vi "CSM_creep_function.vi"() -> ()   [LabVIEW 2009]
doc: "This is the sample data playback waveform and data logging example program. Sample data points are generated using MX Sample Data Array Generator.vi. You will need to replace this VI with your own code. New sample data is sent to the controller each time a status message is recieved from the controller that the next random buffer is running.\nThis program also shows you how to use Active X events. These are used to notify the program when a data buffer is ready for collection and when to load a new buffer of sample data points. Two separate event queues are used: one for data logging and the other for general status, such as when a sample data point buffer can be sent to the controller. Each event handler must run in parallel loops as execution passes to MX Handle Status Change Event.vi and MX Handle Data Ready Event.vi and will not come out of them until an event is received from the console program. When modifiying this example for your own use you may want to setup a third loop to be doing other processing, or you could add code to manipulate the data buffer in the data monitoring loop."
panel:
  in  "Maximum Value":dbl[](array[numeric]) format="%.2f"
  out "Units Strings":string[](array[string])
  in  "Control Modes":u16[](array[ring])=[0, 0, 0, 0] items=["Channel 1", "Channel 2", "Channel 3", "Channel 4"]
  out "Waveform Graph":dbl[][](graph)
  in  "Number of Columns":i32[](array[numeric])
  in  "Interval/Buffer Parameters":T1={"Sample interval - ms (2)"=2.0, "Buffer Length (1000)"=1000, "No. of Buffers (0)"=0} {"Sample interval - ms (2)" min=0.2 format="%.1f"}
  in  "Column Types":i32[][](array[ring])=[[0, 0, 0, 0, 0, 0, 0, 0]] items=["Feedback", "Direct Auxillary"]
  in  "Column Channels":i32[][](array[numeric])=[[1, 1, 1, 1, 1, 1, 1, 1]] min=0 max=200
  in  "Start/Stop":bool
  in  "Axis Selector":i32[](listbox)
  # "Axis 1\nAxis 2\nAxis 3\nAxis 4"
  # "Axis 1\nAxis 2\nAxis 3\nAxis 4"
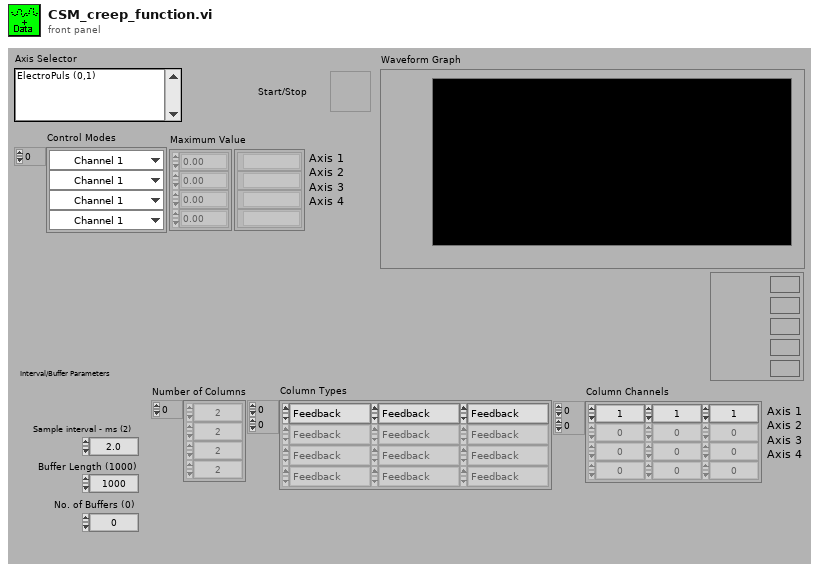
[diagram p1: front panel]
types:
  T1 = cluster{"Sample interval - ms (2)":dbl, "Buffer Length (1000)":i32, "No. of Buffers (0)":i32}
  T2 = cluster{"Name":string, "Type":i32, "SI Full Scale":dbl, "Full Scale":dbl, "Units String":string, "Display Format":string, "Gauge Length":dbl}[][]
  T3 = cluster{"Device ID":i32, "Device Name":string, "Device Type":i32}[]
  T4 = cluster{"Data Sample Format (0)":i8, "Loop code (2)":i8, "Target Amplitude (32767)":i16, "Playback rate":dbl, "Playback Scale":dbl[], "Envelope Ramp Rate":dbl, "Filter Order (0)":i8, "Filter Type (0)":i8, "Filter Bandwidth":dbl}
  T5 = typedef "System Status Reports.ctl" = enum16{"Not this device", "Not Recognised", "Ramp Stopped", "Ramp Running", "Ramp Held", "Random Stopped", "Random Held", "Load Random", "Load Sample", "Sample Playback Held", "Sample Playback Stop - Buffer Underrun", "Sample Playback Continuing", "Returning - EM Frame", "Error Trip", "Segment Counter Trip", "Cycle Counter Trip", "Limit Trip", "Cyclic Stopped", "Cyclic running", "Cyclic Held", "Cyclic Finishing", "Analogue Event 1 tripped", "Analogue Event 2 tripped", "Analogue Event 3 tripped", "Analogue Event 4 tripped", "Analogue Event Off, prepared, armed", "Digital Event Tripped", "Digital Event Off, Prepared, Armed", "Grips Open", "Crosshead Unclamped", "Pump Power Off", "Actuator not Active", "Fault", "Calibrated", "Calibration/Balance in progress", "Console Stop Button Pressed", "Control mode change", "Set Point Change", "Transducer Over-ranged", "GPIB Trigger Armed", "GPIB Trigger Tripped", "Group Trigger Event Tripped", "Trimodal Control Saturated", "Trimodal Control Peak Error", "Trimodal Peak Not Updating", "Digital Line Low", "Digital Line High", "Transducer Disconnected", "Transducer Connected", "Data Logger Idle", "Data Logger Stopped", "Data Logger Started", "Data Logger Data Overrun", "Sample Data Playback Event Tripped", "Next Control Mode Change", "Autotune Completed OK", "Autotune Failed", "Motor Maximum Power Exceeded", "Motor Maximum Temperature Too High", "Motor Maximum Power & Temp too high", "Button Pressed - Function 1", "Button Pressed - Function 2", "Button Pressed - Specimen Protect", "Button Pressed - Reset Gauge Length", "Button Pressed - Return", "Button Pressed - Stop", "Button Pressed - Start", "1st Tensile Travel Limit Tripped", "1st Compressive Travel Limit Tripped", "2nd Tensile Travel Limit Tripped", "2nd Compressive Travel Limit Tripped", "Frame Relay Power Fault - EM", "Emergency Stop - EM", "Drive Disabled - EM", "Power Amp Fault - EM", "Motor Over-Temperature Fault - EM", "Top Grip Open - EM", "Bottom Grip Open - EM", "Interlock Active - EM", "PIP Button Pushed - EM", "Close Grip Request - EM", "High Clutch Active - EM", "Crosshead Moving - EM"}
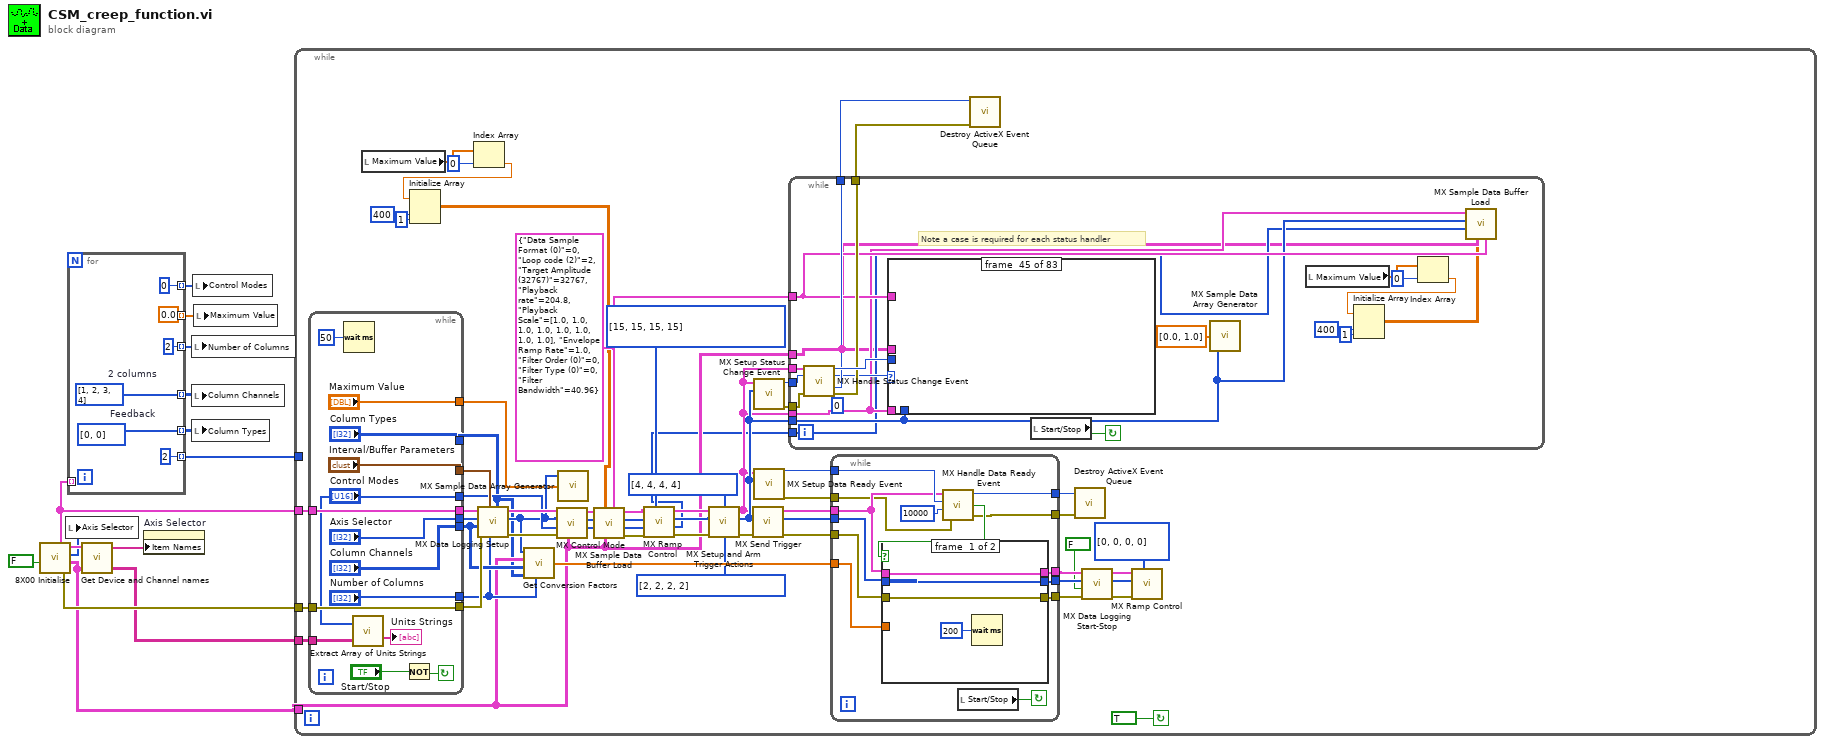
[diagram p0: block diagram]
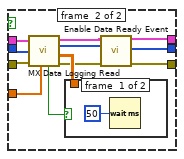
[diagram p2: hidden frame]
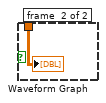
[diagram p3: hidden frame]
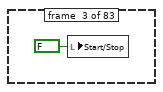
[diagram p6: hidden frame]
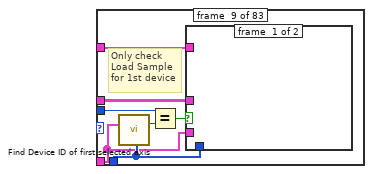
[diagram p12: hidden frame]
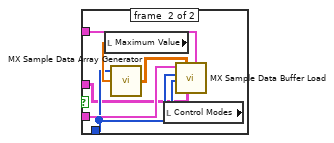
[diagram p13: hidden frame]
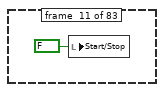
[diagram p15: hidden frame]
diagram:
  n1 = call "8X00 Initialise.vi"("Reset?"=FALSE ("Reset")) -> ("error out"=w12:errorcluster, "Channel Data"=w9:T2, "Axis Selector"=w2:i32[], "Axis Information"=w7:T3)  [unwired: 3 in]
  n2 = local write "Axis Selector"(w2) -> ()
  n3 = for {
    tunnel: w7 -> [_] mode=indexing
    tunnel: [w19] -> w11 mode=indexing
    tunnel: [w18] -> w10 mode=indexing
    tunnel: [2] -> w8 mode=indexing
    tunnel: [2] -> w5 mode=indexing
    tunnel: [0.0] -> w4 mode=indexing
    tunnel: [0] -> w3 mode=indexing
    w18 = i32[] [0, 0]  # Feedback
    w19 = i32[] [1, 2, 3, 4]  # 2 columns
  }
  n4 = call "Get Device and Channel names.vi"("Axis Information"=w7, "Channel Data"=w9) -> ("Device Names"=w13:string[], "Units Strings"=w6:string[][])  [unwired: 1 out]
  n5 = property on="Axis Selector" class="ListBox (strict)"("Item Names"=w13) -> ()  [unwired: 2 in, 2 out]
  n6 = local write "Number of Columns"(w5) -> ()
  n7 = local write "Column Channels"(w11) -> ()
  n8 = local write "Column Types"(w10) -> ()
  n9 = local write "Control Modes"(w3) -> ()
  n10 = local write "Maximum Value"(w4) -> ()
  n11 = while {
    tunnel: w6 -> [w44]
    tunnel: w8 -> [_]
    tunnel: w9 -> [w29]
    tunnel: w7 -> [w75]
    tunnel: w12 -> [w78]
    stop <- TRUE continue-if-true
    w28 = T4 {"Data Sample Format (0)"=0, "Loop code (2)"=2, "Target Amplitude (32767)"=32767, "Playback rate"=204.8, "Playback Scale"=[1.0, 1.0, 1.0, 1.0, 1.0, 1.0, 1.0, 1.0], "Envelope Ramp Rate"=1.0, "Filter Order (0)"=0, "Filter Type (0)"=0, "Filter Bandwidth"=40.96} ("Sample Data Playback Definition")
    w36 = u16[] [0, 0, 0, 0] items=["Stop", "Start or continue", "Hold", "Continue", "Return ramp to set level at fixed rate", "Reserved", "Reserved", "Start Random without demand hold", "Start Random with demand hold", "Prepare Random Start without demand hold", "Prepare Random Start with demand hold", "Unslave", "Reserved", "Reserved", "Start Sample Data Playback or Resume", "Prepare for Start of Sample Data", "Reserved", "Reserved", "Resume Playback"] ("Ramp Control")
    w40 = u16[] [15, 15, 15, 15] items=["Stop", "Start or continue", "Hold", "Continue", "Return ramp to set level at fixed rate", "Reserved", "Reserved", "Start Random without demand hold", "Start Random with demand hold", "Prepare Random Start without demand hold", "Prepare Random Start with demand hold", "Unslave", "Reserved", "Reserved", "Start Sample Data Playback or Resume", "Prepare for Start of Sample Data", "Reserved", "Reserved", "Resume Playback"] ("Ramp Control")
    w61 = u16[] [2, 2, 2, 2] items=["None", "Stop Data Logging", "Start Data Logging"] ("Remote Trigger Action - Data Logging")
    w66 = u16[] [4, 4, 4, 4] items=["None", "Actuator Off", "Stop Waveform", "Hold Waveform", "Transfer", "Log Data Point", "Reset Waveform"] ("Remote Trigger Action")
    # "Note a case is required for each status handler"
    n12 = while {
      tunnel: ["Maximum Value"] -> w42
      tunnel: w44 -> [w83]
      tunnel: ["Control Modes"] -> w45
      tunnel: ["Number of Columns"] -> w72
      tunnel: ["Interval/Buffer Parameters"] -> w76
      tunnel: ["Column Types"] -> w27
      tunnel: [w91] -> w77
      tunnel: w78 -> [w91]
      tunnel: ["Column Channels"] -> w74
      tunnel: ["Axis Selector"] -> w79
      tunnel: [w94] -> w80
      tunnel: w75 -> [w94]
      stop <- w90 continue-if-true
      n13 = Wait (ms)(milliseconds to wait=u32 50) -> ()  [unwired: 1 out]
      n14 = call "Extract Array of Units Strings.vi"("Axes Units Strings"=w83, "Control Modes"="Control Modes") -> ("Units Strings"=→"Units Strings":string[])
      n15 = Not(x="Start/Stop") -> (.not. x?=w90:bool)
    }
    n16 = local read "Maximum Value"() -> (w23:dbl[])
    n17 = Index Array(array=w23, index=0) -> (element=w22:dbl)
    n18 = Initialize Array(w22, 400 ("dimension size"), 1 ("dimension size")) -> (w20:dbl[][])
    n19 = call "MX Data Logging Setup.vi"("Column Types"=w27, "Number of Columns"=w72, "Interval/Buffer Parameters"=w76, "error in (no error)"=w77, "Column Channels"=w74, "Axis Selector"=w79, "Axis Information"=w80) -> ("error out"=w50:errorcluster, "Axis Selector copy"=w43:i32[], "Axis Information out"=w49:T3)  [unwired: 1 out]
    n20 = call "Get Conversion Factors.vi"("Axis Selector"=w43, "Channel Data"=w29, "Column Channels"=w74, "Column Types"=w27, "Number of Columns"=w72) -> ("Conversion Factors"=w73:dbl[])
    n21 = call "MX Control Mode.vi"("Channel Data"=w29, "error in (no error)"=w50, "Control Modes"=w45, "Axis Selector"=w43, "Axis Information"=w49) -> ("Control Modes out"=w46:u16[], "Axis Selector out"=w47:i32[], "Axis Information out"=w48:T3)  [unwired: 1 in, 1 out]
    n22 = call "MX Sample Data Array Generator.vi"("Maximum Value"=w42, "Axis Selector"=w43) -> ()  [unwired: 1 in, 1 out]
    n23 = call "MX Sample Data Buffer Load.vi"("Sample Data Playback Definition"=w28, "Channel Data"=w29, "Sample Data"=w20, "Channels In"=w46, "Axis Selector In"=w47, "Axis Information In"=w48) -> ("error out"=w52:errorcluster, "Channels Out"=w41:u16[], "Axis Selector Out"=w54:i32[], "Axis Information Out"=w56:T3)  [unwired: 2 in]
    n24 = call "MX Ramp Control.vi"("Ramp Control"=w40, "error in (no error)"=w52, "Channels In"=w41, "Axis Selector In"=w54, "Axis Information In"=w56) -> ("error out"=w51:errorcluster, "Channels Out"=w26:u16[], "Axis Selector Out"=w53:i32[], "Axis Information Out"=w55:T3)  [unwired: 2 in]
    n25 = call "MX Setup and Arm Trigger Actions.vi"("Remote Trigger Action"=w66, "Axis Information In"=w55, "Axis Selector"=w53, "Remote Trigger Action - Data Logging"=w61, "error in (no error)"=w51) -> ("Axis Information Out"=w30:T3, "Axis Selector copy"=w33:i32[], "error out"=w62:errorcluster)  [unwired: 2 in]
    n26 = call "MX Send Trigger.vi"("error in (no error)"=w62, "Axis Selector"=w33, "Axis Information"=w30) -> ("error out"=w64:errorcluster, "Axis Selector copy"=w63:i32[], "Axis Information out"=w65:T3)  [unwired: 2 in]
    n27 = call "MX Setup Status Change Event.vi"("Axis Selector"=w33, "Axis Information"=w30) -> ("error out"=w34:errorcluster, "Event Queue"=w35:u32)  [unwired: 6 in]
    n28 = call "MX Setup Data Ready Event.vi"("Axis Selector"=w33, "Axis Information"=w30) -> ("Error Out"=w59:errorcluster, "Event Queue"=w60:u32)  [unwired: 6 in]
    n29 = while {
      tunnel: w28 -> [w137]
      tunnel: w29 -> [w133]
      tunnel: w30 -> [w135]
      tunnel: [w142] -> w31
      tunnel: [w143] -> w32
      tunnel: w33 -> [w136]
      tunnel: w34 -> [w145]
      tunnel: w35 -> [w146]
      tunnel: w30 -> [w141]
      tunnel: w26 -> [w134]
      stop <- w147 continue-if-true
      (unwired) 0 ("index")
      n30 = call "MX Handle Status Change Event.vi"("Axis Information"=w141, "Event Queue"=w146, "Error in (no error)"=w145) -> ("Device ID"=w144:i32, "System Status"=w140:T5, "Event Queue(out)"=w143:i32, "Error out"=w142:errorcluster)  [unwired: 8 in, 1 out]
      n31 = case shown="\"Load Sample\"" w140 {
        tunnel: w144 -> [_ _ _ _ _ _ _ _ w154 _ _ _ _ _ _ _ _ _ _ _ _ _ _ _ _ _ _ _ _ _ _ _ _ _ _ _ _ _ _ _ _ _ _ _ _ _ _ _ _ _ _ _ _ _ _ _ _ _ _ _ _ _ _ _ _ _ _ _ _ _ _ _ _ _ _ _ _ _ _ _ _ _ _]
        tunnel: w136 -> [_ _ _ _ _ _ _ _ w155 _ _ _ _ _ _ _ _ _ _ _ _ _ _ _ _ _ _ _ _ _ _ _ _ _ _ _ _ _ _ _ _ _ _ _ _ _ _ _ _ _ _ _ _ _ _ _ _ _ _ _ _ _ _ _ _ _ _ _ _ _ _ _ _ _ _ _ _ _ _ _ _ _ _]
        tunnel: w135 -> [_ _ _ _ _ _ _ _ w151 _ _ _ _ _ _ _ _ _ _ _ _ _ _ _ _ _ _ _ _ _ _ _ _ _ _ _ _ _ _ _ _ _ _ _ _ _ _ _ _ _ _ _ _ _ _ _ _ _ _ _ _ _ _ _ _ _ _ _ _ _ _ _ _ _ _ _ _ _ _ _ _ _ _]
        tunnel: w133 -> [_ _ _ _ _ _ _ _ w150 _ _ _ _ _ _ _ _ _ _ _ _ _ _ _ _ _ _ _ _ _ _ _ _ _ _ _ _ _ _ _ _ _ _ _ _ _ _ _ _ _ _ _ _ _ _ _ _ _ _ _ _ _ _ _ _ _ _ _ _ _ _ _ _ _ _ _ _ _ _ _ _ _ _]
        tunnel: w137 -> [_ _ _ _ _ _ _ _ w149 _ _ _ _ _ _ _ _ _ _ _ _ _ _ _ _ _ _ _ _ _ _ _ _ _ _ _ _ _ _ _ _ _ _ _ _ _ _ _ _ _ _ _ _ _ _ _ _ _ _ _ _ _ _ _ _ _ _ _ _ _ _ _ _ _ _ _ _ _ _ _ _ _ _]
        frame #0 {
        }
        frame #1 {
        }
        frame #2 {
          n32 = local write "Start/Stop"(FALSE ("Start/Stop")) -> ()
        }
        frame #3 {
        }
        frame #4 {
        }
        frame #5 {
        }
        frame #6 {
        }
        frame #7 {
        }
        frame #8 {
          # "Only check Load Sample for 1st device"
          n33 = call "Find Device ID of first selected axis.vi"("Axis Selector"=w155, "Axis Information"=w151) -> ("Device ID"=w153:i32)
          n34 = Equal?(x=w154, y=w153) -> (x = y?=w152:bool)
          n35 = case shown="True" w152 {
            tunnel: w155 -> [_ w159]
            tunnel: w151 -> [_ w160]
            tunnel: w150 -> [_ w157]
            tunnel: w149 -> [_ w156]
            frame #0 {
            }
            frame #1 {
              n36 = local read "Maximum Value"() -> (w162:dbl[])
              n37 = call "MX Sample Data Array Generator.vi"("Maximum Value"=w162, "Axis Selector"=w159) -> ("Array"=w161:dbl[][])  [unwired: 1 in]
              n38 = local read "Control Modes"() -> (w158:u16[])
              n39 = call "MX Sample Data Buffer Load.vi"("Sample Data Playback Definition"=w156, "Channel Data"=w157, "Sample Data"=w161, "Channels In"=w158, "Axis Selector In"=w159, "Axis Information In"=w160) -> ()  [unwired: 2 in, 4 out]
            }
          }
        }
        frame #9 {
        }
        frame #10 {
          n40 = local write "Start/Stop"(FALSE ("Start/Stop")) -> ()
        }
        frame #11 {
        }
        frame #12 {
        }
        frame #13 {
        }
        frame #14 {
        }
        frame #15 {
        }
        frame #16 {
          n41 = local write "Start/Stop"(FALSE ("Start/Stop")) -> ()
        }
        frame #17 {
        }
        frame #18 {
        }
        frame #19 {
        }
        frame #20 {
        }
        frame #21 {
        }
        frame #22 {
        }
        frame #23 {
        }
        frame #24 {
        }
        frame #25 {
        }
        frame #26 {
        }
        frame #27 {
        }
        frame #28 {
        }
        frame #29 {
        }
        frame #30 {
        }
        frame #31 {
        }
        frame #32 {
        }
        frame #33 {
        }
        frame #34 {
        }
        frame #35 {
          n42 = local write "Start/Stop"(FALSE ("Start/Stop")) -> ()
        }
        frame #36 {
        }
        frame #37 {
        }
        frame #38 {
        }
        frame #39 {
        }
        frame #40 {
        }
        frame #41 {
        }
        frame #42 {
        }
        frame #43 {
        }
        frame #44 {
        }
        frame #45 {
        }
        frame #46 {
        }
        frame #47 {
        }
        frame #48 {
        }
        frame #49 {
        }
        frame #50 {
        }
        frame #51 {
        }
        frame #52 {
        }
        frame #53 {
        }
        frame #54 {
        }
        frame #55 {
        }
        frame #56 {
        }
        frame #57 {
        }
        frame #58 {
        }
        frame #59 {
        }
        frame #60 {
        }
        frame #61 {
        }
        frame #62 {
        }
        frame #63 {
        }
        frame #64 {
        }
        frame #65 {
        }
        frame #66 {
        }
        frame #67 {
        }
        frame #68 {
        }
        frame #69 {
        }
        frame #70 {
        }
        frame #71 {
        }
        frame #72 {
        }
        frame #73 {
        }
        frame #74 {
        }
        frame #75 {
        }
        frame #76 {
        }
        frame #77 {
        }
        frame #78 {
        }
        frame #79 {
        }
        frame #80 {
        }
        frame #81 {
        }
        frame #82 {
        }
      }
      n43 = local read "Start/Stop"() -> (w147:bool)
      n44 = call "MX Sample Data Array Generator.vi"("Maximum Value"=dbl[] [0.0, 1.0], "Axis Selector"=w136) -> ()  [unwired: 1 in, 1 out]
      n45 = local read "Maximum Value"() -> (w129:dbl[])
      n46 = Index Array(array=w129, index=0) -> (element=w128:dbl)
      n47 = Initialize Array(w128, 400 ("dimension size"), 1 ("dimension size")) -> (w132:dbl[][])
      n48 = call "MX Sample Data Buffer Load.vi"("Sample Data Playback Definition"=w137, "Channel Data"=w133, "Sample Data"=w132, "Channels In"=w134, "Axis Selector In"=w136, "Axis Information In"=w135) -> ()  [unwired: 2 in, 4 out]
      n49 = call "MX Sample Data Array Generator.vi"() -> ("Array"=w139:dbl[][])  [unwired: 3 in]
      n50 = call "MX Sample Data Buffer Load.vi"("Sample Data"=w139) -> ()  [unwired: 7 in, 4 out]
    }
    n51 = while {
      tunnel: [w98] -> w57
      tunnel: [w99] -> w58
      tunnel: w59 -> [w95]
      tunnel: w60 -> [w102]
      tunnel: [w103] -> w69
      tunnel: [w104] -> w70
      tunnel: [w105] -> w71
      tunnel: w64 -> [w106]
      tunnel: w73 -> [w107]
      tunnel: w63 -> [w97]
      tunnel: w65 -> [w96]
      stop <- w108 continue-if-true
      n52 = call "MX Handle Data Ready Event.vi"("error in"=w95, "ms timeout (-1)"=10000, "Event Queue"=w102, "Axis Information"=w96) -> ("error out"=w98:errorcluster, "Data Ready?"=w100:bool, "Event Queue(out)"=w99:i32)
      n53 = case shown="True" w100 {
        tunnel: w96 -> [w112 w124]
        tunnel: w97 -> [w111 w123]
        tunnel: w107 -> [_ w122]
        tunnel: w106 -> [w110 w121]
        tunnel: [w112 w115] -> w105
        tunnel: [w111 w116] -> w104
        tunnel: [w110 w117] -> w103
        frame #0 {
          n54 = Wait (ms)(milliseconds to wait=u32 200) -> ()  [unwired: 1 out]
        }
        frame #1 {
          n55 = call "MX Data Logging Read.vi"("Axis Information"=w124, "Axis Selector"=w123, "error in (no error)"=w121, "Conversion Values (100)"=w122) -> ("Axis Information copy"=w113:T3, "Axis Selector copy"=w114:i32[], "Data Available"=w120:bool, "Collected Data - Eng Units"=w119:dbl[][], "error out"=w118:errorcluster)  [unwired: 2 out]
          n56 = case shown="True" w120 {
            tunnel: w119 -> [_ w126]
            frame #0 {
              n57 = Wait (ms)(milliseconds to wait=u32 50) -> ()  [unwired: 1 out]
            }
            frame #1 {
              "Waveform Graph" <- w126
            }
          }
          n58 = call "Enable Data Ready Event.vi"("Axis Information"=w113, "Axis Selector"=w114, "Error (No Error)"=w118) -> ("Axis Information Out"=w115:T3, "Axis Selector Out"=w116:i32[], "Error Out"=w117:errorcluster)  [unwired: 10 in]
        }
      }
      n59 = local read "Start/Stop"() -> (w108:bool)
    }
    n60 = call <vilib>:"Destroy ActiveX Event Queue.vi"("error in (no error)"=w31, "Event Queue"=w32) -> ()  [unwired: 5 in, 1 out]
    n61 = call <vilib>:"Destroy ActiveX Event Queue.vi"("error in (no error)"=w57, "Event Queue"=w58) -> ()  [unwired: 5 in, 1 out]
    n62 = call "MX Data Logging Start-Stop.vi"("error in (no error)"=w69, "Start (T)"=FALSE, "Axis Selector"=w70, "Axis Information"=w71) -> ("error out"=w38:errorcluster, "Axis Selector copy"=w37:i32[], "Axis Information out"=w39:T3)  [unwired: 4 in]
    n63 = call "MX Ramp Control.vi"("Ramp Control"=w36, "error in (no error)"=w38, "Axis Selector In"=w37, "Axis Information In"=w39) -> ()  [unwired: 3 in, 4 out]
  }
